vi "Construct pyWebscraper Command.vi"(7 "pyWebscraper Test Type":T2, 8 "error in (no error)":errorcluster, 9 "Image Configuration":T1={"Images"=[], "Confidence"=0.9} caption="Image Configuration (Only applicable for ratio test)" {"Confidence" min=0.0 max=1.0 format="%.2g"}, 10 "pyWebscraper Configuration":T3={"URL"="", "Delay (s)"=10} {"Delay (s)" max=1}) -> (0 "error out":errorcluster, 2 "pyWebscraper Command":string)   [LabVIEW 2016, in "Webscraper.lvlib"]
doc: "This VI sends \"-openprj<FILENAME> -open<FILENAME>[,<SADDR>] -auto -exit\" command to JFlash.exe CLI to erase, program and verify the flash. \n\nNote: The parameter Address apply only if the data file is a *.bin file or *.c file."
uses:
  Webscraper.lvlib
  Type Definitions/pyWebscraper Configuration.ctl
  Type Definitions/pyWebscraper Test Type.ctl
  Type Definitions/pyWebscraper Image Configuration.ctl
  Type Definitions/pyWebscraper ArgParse Type.ctl
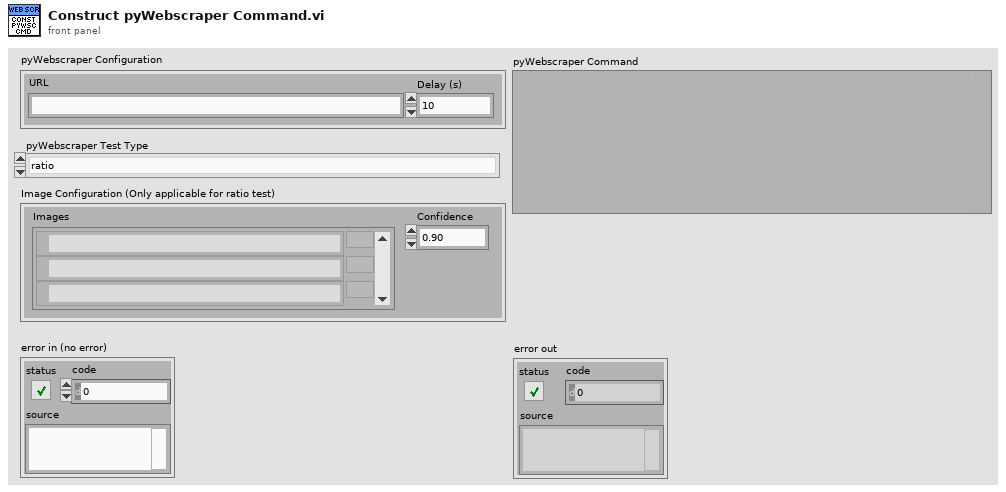
[diagram p1: front panel]
types:
  T1 = typedef "Webscraper.lvlib/pyWebscraper Image Configuration.ctl" = cluster{"Images":path[], "Confidence":dbl}
  T2 = typedef "Webscraper.lvlib/pyWebscraper Test Type.ctl" = enum16{"ratio", "overview", "livepara", "counts", "maxvalue", "alarm_ph2", "nwconfig"}
  T3 = typedef "Webscraper.lvlib/pyWebscraper Configuration.ctl" = cluster{"URL":string, "Delay (s)":u32}
  T4 = typedef "Webscraper.lvlib/pyWebscraper ArgParse Type.ctl" = enum16{"url", "test", "image", "confidence", "delay"}
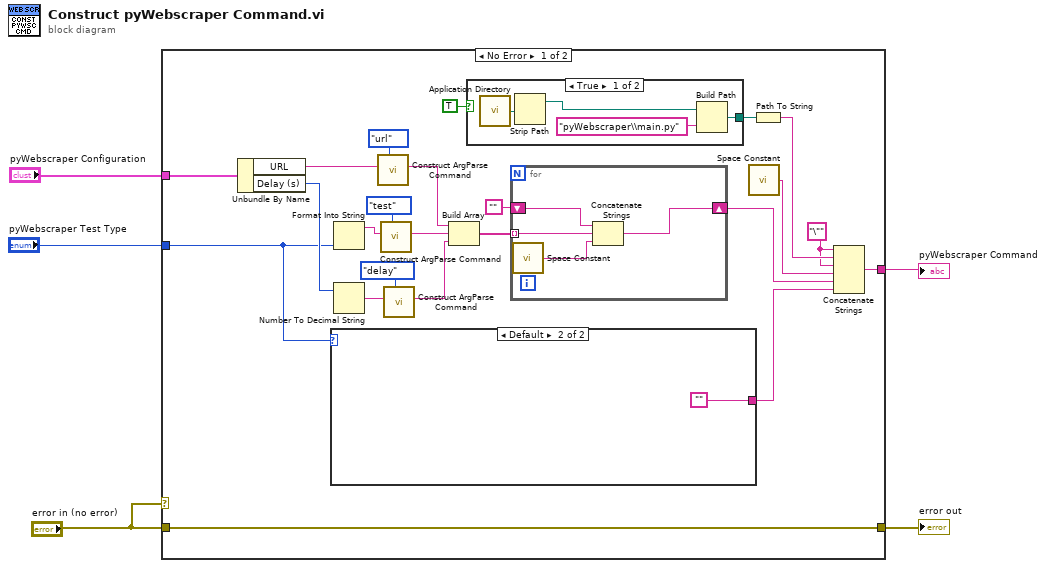
[diagram p0: block diagram]
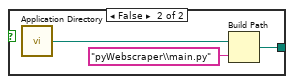
[diagram p2: hidden frame]
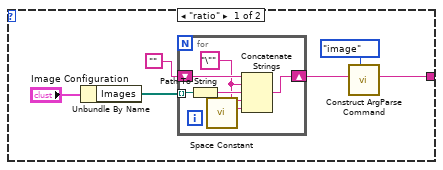
[diagram p3: hidden frame]
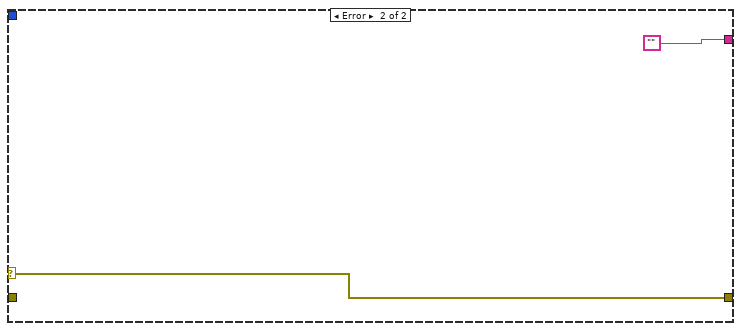
[diagram p4: hidden frame]
diagram:
  n1 = case shown="No Error" "error in (no error)" {
    selector: "error in (no error)" -> [_ w54]
    tunnel: [w8 w54] -> w5
    tunnel: [w15 ""] -> w4
    tunnel: "pyWebscraper Configuration" -> [w28 _]
    tunnel: "pyWebscraper Test Type" -> [w9 _]
    tunnel: "error in (no error)" -> [w8 _]
    frame No Error {
      w7 = "\""
      n2 = Unbundle By Name(w28) -> ("URL"=w26:string, "Delay (s)"=w10:u32)
      n3 = case shown="Default" w9 {
        tunnel: [w41 ""] -> w16
        frame "ratio" {
          n4 = Unbundle By Name("Image Configuration") -> ("Images"=w45:path[])
          n5 = for {
            tunnel: w45 -> [w51] mode=indexing
            shift-right: [w48] -> w42
            shift-left: "" -> [w47]
            w46 = "\"" ("string")
            n6 = Path To String(path=w51) -> (string=w50:string)
            n7 = call <vilib>:"Space Constant.vi"() -> ("String"=w49:string)
            n8 = Concatenate Strings(w47, w46, w50, w46, w49) -> (w48:string)
          }
          n9 = call "Construct ArgParse Command.vi"("pyWebscraper ArgParse Command Type"=pyWebscraper_ArgParse_Type."image", "Input"=w42) -> ("Output"=w41:string)  [unwired: 8 in, 1 out]
        }
        frame Default {
        }
      }
      n10 = Format Into String(w9) -> (resulting string=w24:string)  [unwired: 3 in, 1 out]
      n11 = Number To Decimal String(number=w10) -> (decimal integer string=w22:string)  [unwired: 1 in]
      n12 = call "Construct ArgParse Command.vi"("pyWebscraper ArgParse Command Type"=pyWebscraper_ArgParse_Type."url", "Input"=w26) -> ("Output"=w21:string)  [unwired: 8 in, 1 out]
      n13 = call "Construct ArgParse Command.vi"("pyWebscraper ArgParse Command Type"=pyWebscraper_ArgParse_Type."test", "Input"=w24) -> ("Output"=w20:string)  [unwired: 8 in, 1 out]
      n14 = call "Construct ArgParse Command.vi"("pyWebscraper ArgParse Command Type"=pyWebscraper_ArgParse_Type."delay", "Input"=w22) -> ("Output"=w19:string)  [unwired: 8 in, 1 out]
      n15 = Build Array(w21, w20, w19) -> (w18:string[])
      n16 = case shown="True" TRUE {
        tunnel: [w31 w34] -> w14
        frame True {
          n17 = call <vilib>:"Application Directory.vi"() -> ("Application Directory"=w30:path)
          n18 = Strip Path(path=w30) -> (stripped path=w29:path)  [unwired: 1 out]
          n19 = Build Path(base path=w29, name or relative path="pyWebscraper\\main.py") -> (appended path=w31:path)
        }
        frame False {
          n20 = call <vilib>:"Application Directory.vi"() -> ("Application Directory"=w33:path)
          n21 = Build Path(base path=w33, name or relative path="pyWebscraper\\main.py") -> (appended path=w34:path)
        }
      }
      n22 = for {
        tunnel: w18 -> [w39] mode=indexing
        shift-right: [w36] -> w17
        shift-left: "" -> [w38]
        n23 = call <vilib>:"Space Constant.vi"() -> ("String"=w37:string)
        n24 = Concatenate Strings(w38, w39, w37) -> (w36:string)
      }
      n25 = call <vilib>:"Space Constant.vi"() -> ("String"=w12:string)
      n26 = Path To String(path=w14) -> (string=w13:string)
      n27 = Concatenate Strings(w7, w13, w7, w12, w17, w16) -> (w15:string)
    }
    frame Error {
    }
  }
  "error out" <- w5
  "pyWebscraper Command" <- w4
